vi "Name.CheckErrors.vi"(9 "ID":u16, 10 "Name":string, 11 "Existing Frames":string[](array[string])) -> (2 "Error?":bool, 3 "Error String":string)   [LabVIEW 2015, in "Diagnostics Addon System Explorer.lvlib"]
uses:
  Diagnostics Addon System Explorer.lvlib
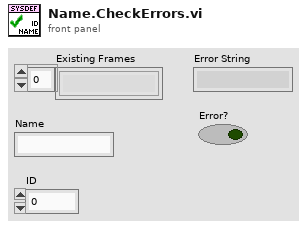
[diagram p1: front panel]
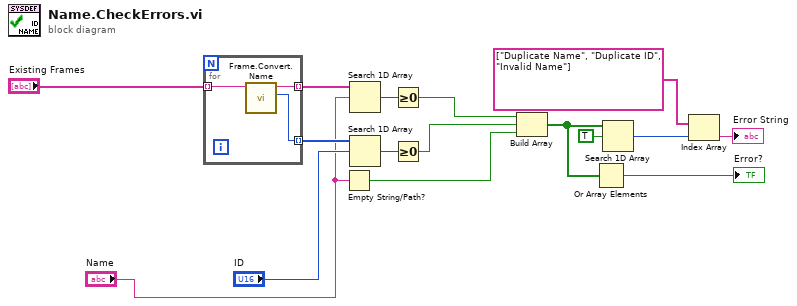
[diagram p0: block diagram]
diagram:
  n1 = for {
    tunnel: "Existing Frames" -> [w19] mode=indexing
    tunnel: [w18] -> w15 mode=indexing
    tunnel: [w17] -> w13 mode=indexing
    n2 = call "Frame.Convert.Name.vi"("VS Frame Name"=w19) -> ("ID"=w18:u16, "Frame Name"=w17:string)  [unwired: 9 in]
  }
  n3 = Empty String/Path?(string/path="Name") -> (empty?=w2:bool)
  n4 = Search 1D Array(1D array=w13, element="Name") -> (index of element=w11:i32)  [unwired: 1 in]
  n5 = Search 1D Array(1D array=w15, element="ID") -> (index of element=w12:i32)  [unwired: 1 in]
  n6 = Greater Or Equal To 0?(x=w11) -> (x >= 0?=w4:bool)
  n7 = Greater Or Equal To 0?(x=w12) -> (x >= 0?=w3:bool)
  n8 = Build Array(w4, w3, w2) -> (w8:bool[])
  n9 = Or Array Elements(Boolean array=w8) -> (logical OR=→"Error?":bool)
  n10 = Search 1D Array(1D array=w8, element=TRUE) -> (index of element=w6:i32)  [unwired: 1 in]
  n11 = Index Array(array=string[] ["Duplicate Name", "Duplicate ID", "Invalid Name"], index=w6) -> (element=→"Error String":string)
